vi "GCentral Temporary Directory--constant.vi"() -> (3 "GCentral Temporary Directory":path)   [LabVIEW 2016, in "WSsupport.lvlib"]
uses:
  WSsupport.lvlib
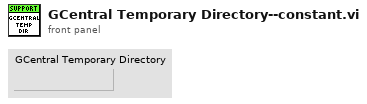
[diagram p1: front panel]
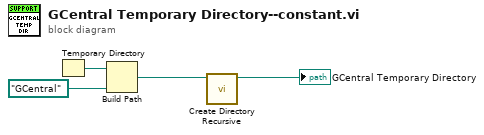
[diagram p0: block diagram]
diagram:
  n1 = Temporary Directory() -> (w4:path)
  n2 = Build Path(base path=w4, name or relative path=path "GCentral") -> (appended path=w2:path)
  n3 = call <vilib>:"Create Directory Recursive.vi"("directory"=w2) -> ("directory copy"=→"GCentral Temporary Directory":path)  [unwired: 4 in, 2 out]
